vi "Read Joystick.vi"(8 "Joystick Deadbanded Value (default of 0.1)":dbl, 11 "Joystick L 1 DevRef":T1) -> (1 "Joystick L 2 X Axis":dbl, 2 "Joystick L 1 Y Axis":dbl, 3 "Joystick L 1 X Axis":dbl)   [LabVIEW 2014]
uses:
  <vilib>/Rock Robotics/WPI/Joystick/WPI_JoystickDevRef.ctl
  <vilib>/Rock Robotics/WPI/Joystick/WPI_JoystickDeviceEnum.ctl
  Global Variables.vi
  <vilib>/Rock Robotics/WPI/Joystick/WPI_JoystickGetSetRefNum.vi
  <vilib>/Utility/file.llb/Write To Spreadsheet File (DBL).vi
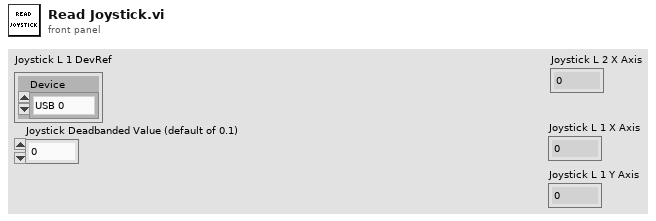
[diagram p1: front panel]
types:
  T1 = typedef "WPI_JoystickDevRef.ctl" = cluster{"Device":T2}
  T2 = typedef "WPI_JoystickDeviceEnum.ctl" = enum16{"USB 0", "USB 1", "USB 2", "USB 3", "USB 4", "USB 5"}
  T3 = cluster{"Buttons[0]":bool, "Buttons[1]":bool, "Buttons[2]":bool, "Buttons[3]":bool, "Buttons[4]":bool, "Buttons[5]":bool, "Buttons[6]":bool, "Buttons[7]":bool, "Buttons[8]":bool}
  T4 = cluster{"Axes[0]":dbl, "Axes[1]":dbl, "Axes[2]":dbl, "Axes[3]":dbl, "Axes[4]":dbl, "Axes[5]":dbl, "Axes[6]":dbl, "Axes[7]":dbl, "Axes[8]":dbl}
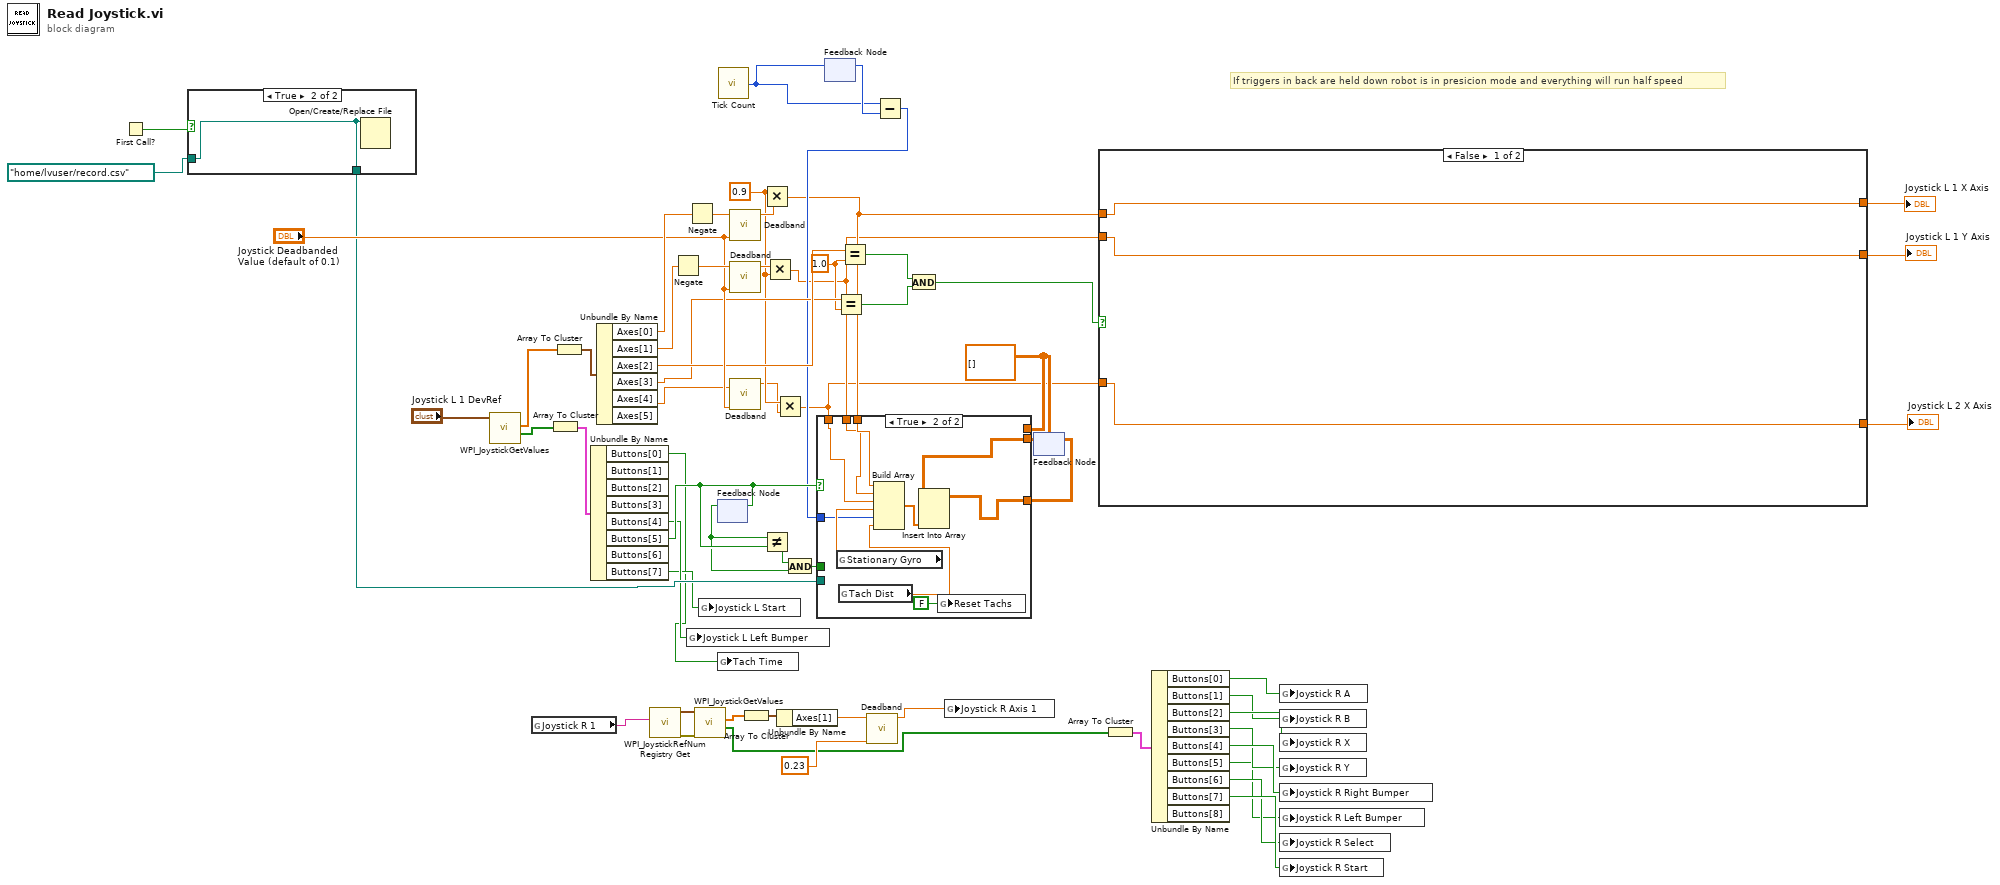
[diagram p0: block diagram]
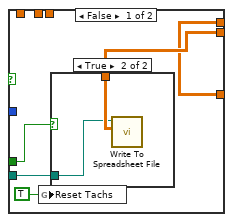
[diagram p3: hidden frame]
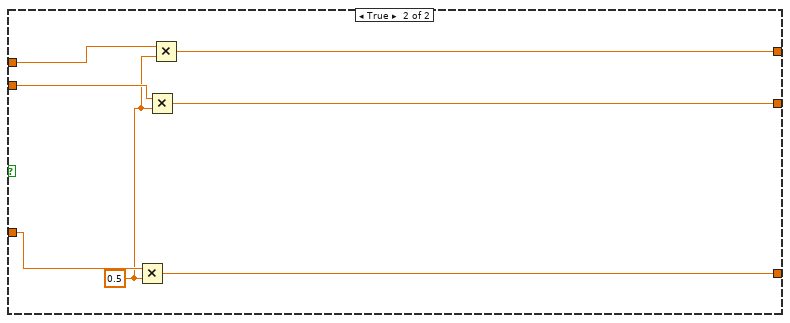
[diagram p5: hidden frame]
diagram:
  w3 = 0.9 ("x")
  w12 = dbl[][] []
  w31 = 1.0 ("y")
  # "If triggers in back are held down robot is in presicion mode and everything will run half speed"
  n1 = First Call?() -> (First Call?: T/F=w18:bool)
  n2 = case shown="True" w18 {
    tunnel: [w62 w63] -> w17
    tunnel: path "/home/lvuser/record.csv" ("file path (use dialog)") -> [w62 w63]
    frame False {
    }
    frame True {
      n3 = Open/Create/Replace File(file path (use dialog)=w63) -> ()  [unwired: 5 in, 3 out]
    }
  }
  n4 = call <vilib>:"WPI_JoystickGetValues.vi"("JoystickDevRef"="Joystick L 1 DevRef") -> ("Buttons"=w58:bool[], "Axes"=w60:dbl[])  [unwired: 6 in, 3 out]
  n5 = global read "Global Variables.vi" "Joystick R 1"() -> (w49:string)
  n6 = Array To Cluster(array=w58) -> (cluster=w57:T3)
  n7 = Array To Cluster(array=w60) -> (cluster=w59:T4)
  n8 = Unbundle By Name(w57) -> ("Buttons[0]"=w8:bool, "Buttons[4]"=w14:bool, "Buttons[5]"=w21:bool, "Buttons[7]"=w13:bool)  [unwired: 4 out]
  n9 = Unbundle By Name(w59) -> ("Axes[0]"=w56:dbl, "Axes[1]"=w53:dbl, "Axes[2]"=w33:dbl, "Axes[3]"=w32:dbl, "Axes[4]"=w34:dbl)  [unwired: 1 out]
  n10 = call <vilib>:"WPI_JoystickRefNum Registry Get.vi"("refnum name"=w49) -> ("error out"=w48:errorcluster, "JoystickDevRef"=w47:T1)  [unwired: 9 in]
  n11 = Negate(x=w53) -> (-x=w54:dbl)
  n12 = Negate(x=w56) -> (-x=w55:dbl)
  n13 = global write "Global Variables.vi" "Joystick L Left Bumper"(w14) -> ()
  n14 = call <vilib>:"WPI_JoystickGetValues.vi"("error in (no error)"=w48, "JoystickDevRef"=w47) -> ("Buttons"=w36:bool[], "Axes"=w50:dbl[])  [unwired: 5 in, 3 out]
  n15 = global write "Global Variables.vi" "Joystick L Start"(w13) -> ()
  n16 = feedback #1() -> (w20:bool)  [unwired: 1 in]
  n17 = feedback-in #1(w21) -> ()
  n18 = global write "Global Variables.vi" "Tach Time"(w8) -> ()
  n19 = call "Tick Count"() -> ("Tick Count(mSec)"=w10:u32)
  n20 = call "Deadband.vi"("Value to Deadband (default of 0.1)"="Joystick Deadbanded Value (default of 0.1)", "Value"=w55) -> ("Deadbanded Value"=w7:dbl)  [unwired: 9 in]
  n21 = call "Deadband.vi"("Value to Deadband (default of 0.1)"="Joystick Deadbanded Value (default of 0.1)", "Value"=w54) -> ("Deadbanded Value"=w5:dbl)  [unwired: 9 in]
  n22 = call "Deadband.vi"("Value to Deadband (default of 0.1)"="Joystick Deadbanded Value (default of 0.1)", "Value"=w34) -> ("Deadbanded Value"=w2:dbl)  [unwired: 9 in]
  n23 = Array To Cluster(array=w50) -> (cluster=w51:T4)
  n24 = Multiply(x=w3, y=w7) -> (x*y=w6:dbl)
  n25 = Not Equal?(x=w20, y=w21) -> (x != y?=w22:bool)
  n26 = Multiply(x=w5, y=w3) -> (x*y=w4:dbl)
  n27 = Multiply(x=w3, y=w2) -> (x*y=w1:dbl)
  n28 = Unbundle By Name(w51) -> ("Axes[1]"=w45:dbl)
  n29 = And(x=w22, y=w20) -> (x .and. y?=w19:bool)
  n30 = feedback-in #2(w10) -> ()
  n31 = feedback #2() -> (w11:u32)  [unwired: 1 in]
  n32 = Equal?(x=w32, y=w31) -> (x = y?=w29:bool)
  n33 = Equal?(x=w33, y=w31) -> (x = y?=w30:bool)
  n34 = call "Deadband.vi"("Value to Deadband (default of 0.1)"=0.23, "Value"=w45) -> ("Deadbanded Value"=w44:dbl)  [unwired: 9 in]
  n35 = Subtract(x=w10, y=w11) -> (x-y=w9:u32)
  n36 = And(x=w30, y=w29) -> (x .and. y?=w28:bool)
  n37 = global write "Global Variables.vi" "Joystick R Axis 1"(w44) -> ()
  n38 = feedback #3(w12) -> (w23:dbl[][])
  n39 = case shown="True" w21 {
    tunnel: w6 -> [_ w78]
    tunnel: [w65 w80] -> w24
    tunnel: w23 -> [w67 w79]
    tunnel: w4 -> [_ w77]
    tunnel: w1 -> [_ w76]
    tunnel: w19 -> [w68 _]
    tunnel: w17 -> [w66 _]
    tunnel: w12 -> [w65 _]
    tunnel: w9 -> [_ w73]
    frame False {
      n40 = global write "Global Variables.vi" "Reset Tachs"(TRUE ("Reset Tachs")) -> ()
      n41 = case shown="True" w68 {
        tunnel: w67 -> [_ w70]
        tunnel: w66 -> [_ w69]
        frame False {
        }
        frame True {
          n42 = call-poly <vilib>:"Write To Spreadsheet File.vi"("2D data"=w70, "file path (dialog if empty)"=w69) -> ()  [unwired: 6 in, 1 out]
        }
      }
    }
    frame True {
      n43 = global read "Global Variables.vi" "Stationary Gyro"() -> (w74:dbl)
      n44 = global read "Global Variables.vi" "Tach Dist"() -> (w72:dbl)
      n45 = Build Array(w78, w77, w76, w74, w73, w72) -> (w75:dbl[])
      n46 = Insert Into Array(array=w79, new element=w75) -> (w80:dbl[][])  [unwired: 2 in]
      n47 = global write "Global Variables.vi" "Reset Tachs"(FALSE ("Reset Tachs")) -> ()
    }
  }
  n48 = feedback-in #3(w24) -> ()
  n49 = case shown="False" w28 {
    tunnel: w1 -> [w81 w90]
    tunnel: w4 -> [w82 w89]
    tunnel: w6 -> [w83 w87]
    tunnel: [w83 w86] -> w27
    tunnel: [w82 w85] -> w26
    tunnel: [w81 w84] -> w25
    frame False {
    }
    frame True {
      w88 = 0.5 ("y")
      n50 = Multiply(x=w90, y=w88) -> (x*y=w84:dbl)
      n51 = Multiply(x=w89, y=w88) -> (x*y=w85:dbl)
      n52 = Multiply(x=w87, y=w88) -> (x*y=w86:dbl)
    }
  }
  "Joystick L 1 Y Axis" <- w26
  "Joystick L 1 X Axis" <- w27
  "Joystick L 2 X Axis" <- w25
  n53 = Array To Cluster(array=w36) -> (cluster=w37:T3)
  n54 = Unbundle By Name(w37) -> ("Buttons[0]"=w35:bool, "Buttons[1]"=w38:bool, "Buttons[2]"=w39:bool, "Buttons[3]"=w40:bool, "Buttons[4]"=w41:bool, "Buttons[5]"=w15:bool, "Buttons[6]"=w42:bool, "Buttons[7]"=w43:bool)  [unwired: 1 out]
  n55 = global write "Global Variables.vi" "Joystick R A"(w35) -> ()
  n56 = global write "Global Variables.vi" "Joystick R B"(w38) -> ()
  n57 = global write "Global Variables.vi" "Joystick R X"(w39) -> ()
  n58 = global write "Global Variables.vi" "Joystick R Y"(w40) -> ()
  n59 = global write "Global Variables.vi" "Joystick R Right Bumper"(w41) -> ()
  n60 = global write "Global Variables.vi" "Joystick R Left Bumper"(w15) -> ()
  n61 = global write "Global Variables.vi" "Joystick R Select"(w42) -> ()
  n62 = global write "Global Variables.vi" "Joystick R Start"(w43) -> ()
